vi "Test_ReadValue_QueueOverflow_ReportDataLost.vi"(8 "error in (no error)":errorcluster, 11 "TestCase in":refnum<class "TestQueueTransport.lvclass">) -> (0 "error out":errorcluster, 3 "TestCase out":refnum<class "TestQueueTransport.lvclass">)   [LabVIEW 2017, in "TestQueueTransport.lvclass"]
uses:
  TestQueueTransport.lvclass
  Source/Concrete/QueueTransport/QueueTransport.lvclass/QueueTransport.ctl
  Source/Concrete/QueueTransport/QueueTransport.lvclass
  C:/Git/composed-transport/Source/ITransport/ITransport.lvclass
  <vilib>/Utility/error.llb/Error Cluster From Error Code.vi
  Source/ITransport/ITransport.lvclass
panel:
  out "Data Lost?":bool
  out "Data":variant
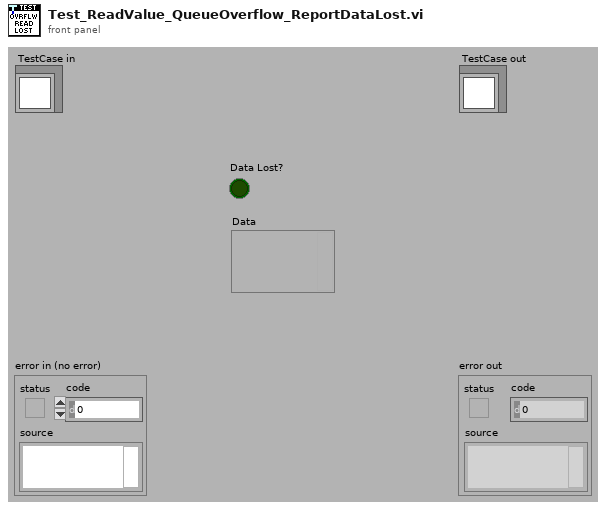
[diagram p1: front panel]
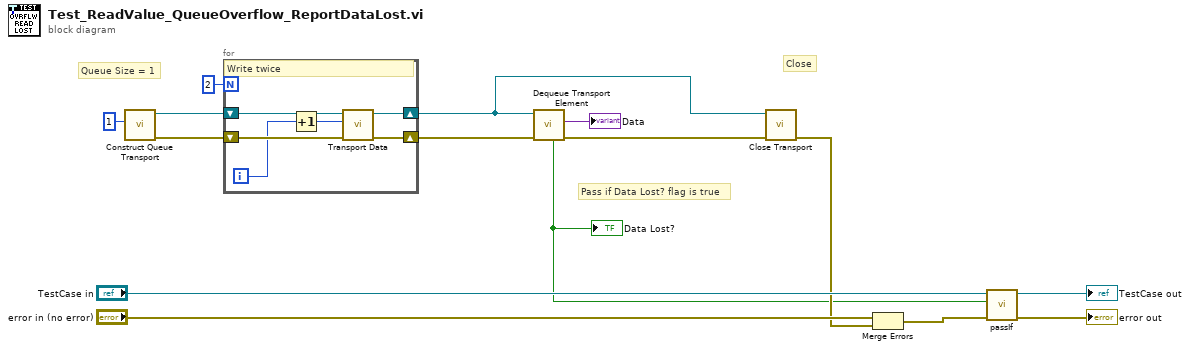
[diagram p0: block diagram]
diagram:
  # "Pass if Data Lost? flag is true"
  # "Queue Size = 1"
  # "Close"
  n1 = call "Construct Queue Transport.vi"("Max Queue Size (-1)"=1) -> ("error out"=w10:errorcluster, "QueueTransport"=w7:refnum<class "QueueTransport.lvclass">)  [unwired: 9 in]
  n2 = for {
    N: 2 -> [_]
    shift-right: [w20] -> w8
    shift-left: w10 -> [w21]
    shift-right: [w18] -> w3
    shift-left: w7 -> [w19]
    i -> [w17]
    # "Write twice"
    n3 = Increment(x=w17) -> (x+1=w16:i32)
    n4 = call "Transport Data.vi"("error in (no error)"=w21, "Value"=w16, "ITransport in"=w19) -> ("error out"=w20:errorcluster, "ITransport out"=w18:refnum<class "QueueTransport.lvclass">)  [unwired: 7 in]
  }
  n5 = call "Dequeue Transport Element.vi"("error in (no error)"=w8, "QueueTransport"=w3) -> ("error out"=w4:errorcluster, "Data"=→"Data":variant, "Data Lost?"=w2:bool)  [unwired: 6 in, 1 out]
  "Data Lost?" <- w2
  n6 = call-dynamic "Close Transport.vi"("error in (no error)"=w4, "QueueTransport"=w3) -> ("error out"=w9:errorcluster)  [unwired: 9 in]
  n7 = Merge Errors("error in (no error)", w9) -> (w11:errorcluster)
  n8 = call-dynamic "passIf.vi"("error in (no error)"=w11, "pass"=w2, "TestCase in"="TestCase in") -> ("error out"=→"error out":errorcluster, "TestCase out"=→"TestCase out":refnum<class "TestQueueTransport.lvclass">)  [unwired: 7 in]
